vi "Delete Dcode Script_c18.vi"() -> (3 "Date Codes":string[](array[string]))   [LabVIEW 2020]
uses:
  MS SQL/MS_Global.vi
panel:
  in  "Column":string="RFID"
  out "spreadsheet string 2":string
  out "date/time string":string
  out "spreadsheet string":string
  out "Time Stamp":timestamp
  out "time stamp":timestamp
  out "Ent_Stamp":timestamp
  out "Date Code":string
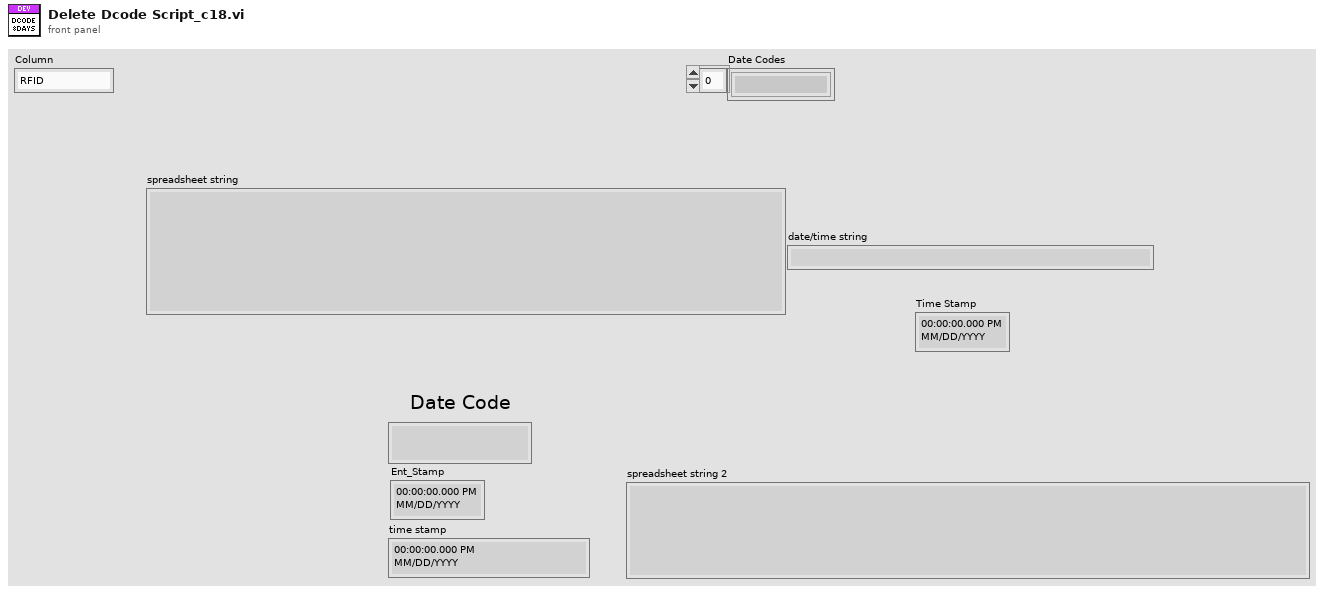
[diagram p1: front panel]
types:
  T1 = typedef "LVDateTimeRec.ctl" = cluster{"fractional second":dbl, "second":i32, "minute":i32, "hour":i32, "day of month":i32, "month":i32, "year":i32, "day of week":i32, "day of year":i32, "DST":i32}
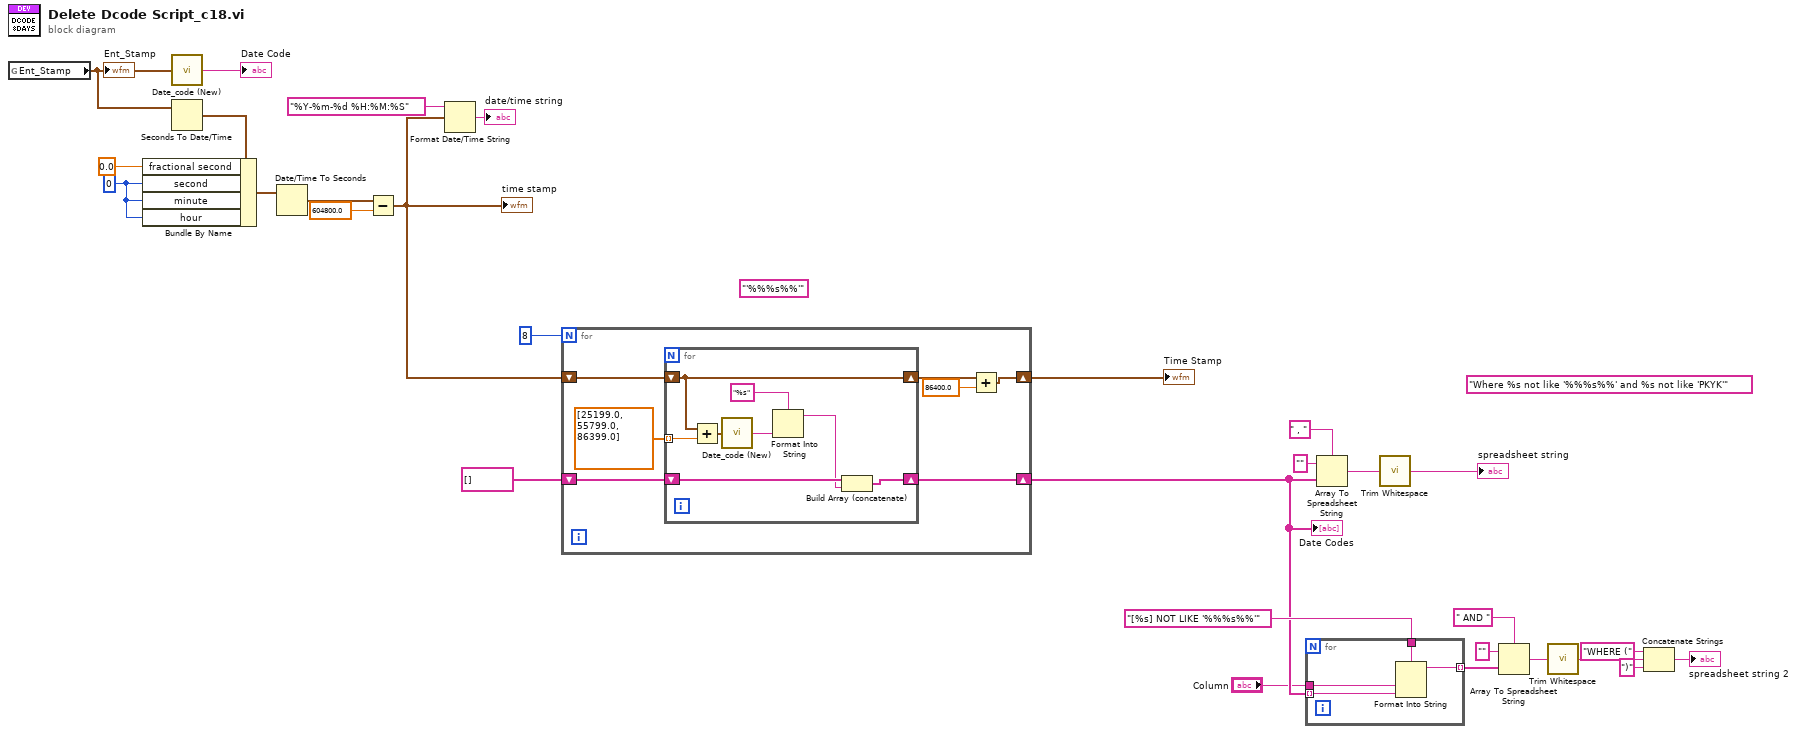
[diagram p0: block diagram]
diagram:
  (unwired) "Where %s not like '%%%s%%' and %s not like 'PKYK'" ("SQL query")
  (unwired) "'%%%s%%'" ("format string")
  w28 = 0 ("second")
  n1 = global read "MS_Global.vi" "Ent_Stamp"() -> (w1:timestamp)
  "Ent_Stamp" <- w1
  n2 = call "Date_code (New).vi"("Date"=w1) -> ("Date Code"=→"Date Code":string)  [unwired: 13 in, 1 out]
  n3 = Seconds To Date/Time(time stamp (now)=w1) -> (date time rec=w26:T1)  [unwired: 1 in]
  n4 = Bundle By Name(cluster=w26, "fractional second"=0.0, "second"=w28, "minute"=w28, "hour"=w28) -> (w25:T1)
  n5 = Date/Time To Seconds(2:w25) -> (0:w24:timestamp)  [unwired: 1 in]
  n6 = Subtract(x=w24, y=604800.0 ("fractional second")) -> (x-y=w14:timestamp)
  "time stamp" <- w14
  n7 = Format Date/Time String(time format string (%c)="%Y-%m-%d %H:%M:%S", seconds (now)=w14) -> (date/time string=→"date/time string":string)  [unwired: 1 in]
  n8 = for {
    N: 8 -> [_]
    shift-right: [w32] -> w20
    shift-left: w14 -> [w31]
    shift-right: [w34] -> w11
    shift-left: string[] [] ("Sorted Array out") -> [w35]
    n9 = for {
      tunnel: dbl[] [25199.0, 55799.0, 86399.0] ("Sorted Array out") -> [w44] mode=indexing
      shift-right: [w42] -> w34
      shift-left: w35 -> [w43]
      shift-right: [w40] -> w30
      shift-left: w31 -> [w40]
      n10 = Add(x=w40, y=w44) -> (x+y=w41:timestamp)
      n11 = call "Date_code (New).vi"("Date"=w41) -> ("Date Code"=w39:string)  [unwired: 13 in, 1 out]
      n12 = Format Into String(format string="%s", w39) -> (resulting string=w38:string)  [unwired: 2 in, 1 out]
      n13 = Build Array (concatenate)(w43, w38) -> (w42:string[])
    }
    n14 = Add(x=w30, y=86400.0) -> (x+y=w32:timestamp)
  }
  "Time Stamp" <- w20
  "Date Codes" <- w11
  n15 = for {
    tunnel: "[%s] NOT LIKE '%%%s%%'" ("SQL query") -> [w48]
    tunnel: "Column" -> [w47]
    tunnel: w11 -> [w46] mode=indexing
    tunnel: [w45] -> w8 mode=indexing
    n16 = Format Into String(format string=w48, w47, w46) -> (resulting string=w45:string)  [unwired: 2 in, 1 out]
  }
  n17 = Array To Spreadsheet String(delimiter (Tab)=" , ", array=w11, 3:"" ("format string")) -> (spreadsheet string=w17:string)
  n18 = call <vilib>:"Trim Whitespace.vi"("string"=w17) -> ("trimmed string"=→"spreadsheet string":string)  [unwired: 1 in]
  n19 = Array To Spreadsheet String(delimiter (Tab)=" AND ", array=w8, 3:"" ("format string")) -> (spreadsheet string=w7:string)
  n20 = call <vilib>:"Trim Whitespace.vi"("string"=w7) -> ("trimmed string"=w5:string)  [unwired: 1 in]
  n21 = Concatenate Strings("WHERE (" ("string"), w5, ")" ("string")) -> (→"spreadsheet string 2":string)
